vi "Compute 1 A-Scan Parameters.vi"(8 "error in (no error)":errorcluster, 10 "Laser In":refnum<class "Laser.lvclass">, 11 "DAQ Class.lvclass":refnum<class "DAQ Class.lvclass">) -> (0 "error out":errorcluster, 2 "DAQ Parameters":T1, 3 "DAQ Class.lvclass 2":refnum<class "DAQ Class.lvclass">)   [LabVIEW 2015, in "DAQ Class.lvclass"]
uses:
  DAQ Class.lvclass
  DAQ Parameters.ctl
  Trigger Source.ctl
  Trigger Slope.ctl
  Type Defs/OCT DAQ Channel Data Type.ctl
  Clock Control.ctl
  Laser/Laser.lvclass
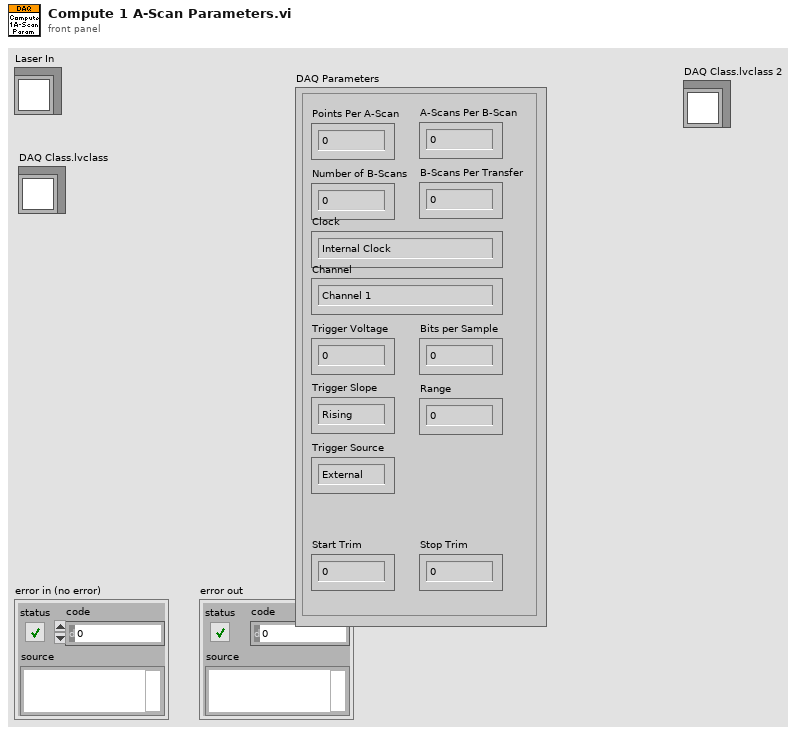
[diagram p1: front panel]
types:
  T1 = typedef "DAQ Class.lvclass/DAQ Parameters.ctl" = cluster{"Points Per A-Scan":u32, "A-Scans Per B-Scan":u32, "Number of B-Scans":u32, "B-Scans Per Transfer":u32, "Trigger Voltage":sgl, "Trigger Source":T2, "Trigger Slope":T3, "Channel":T4, "Clock":T5, "Bits per Sample":dbl, "Range":dbl, "Start Trim":u32, "Stop Trim":u32}
  T2 = typedef "DAQ Class.lvclass/Trigger Source.ctl" = enum16{"External", "Channel A", "Channel B"}
  T3 = typedef "DAQ Class.lvclass/Trigger Slope.ctl" = enum16{"Rising", "Falling"}
  T4 = typedef "OCT DAQ Channel Data Type.ctl" = enum16{"Channel 1", "Channel 2", "Channel 1 and 2"}
  T5 = typedef "DAQ Class.lvclass/Clock Control.ctl" = enum16{"Internal Clock", "External Clock"}
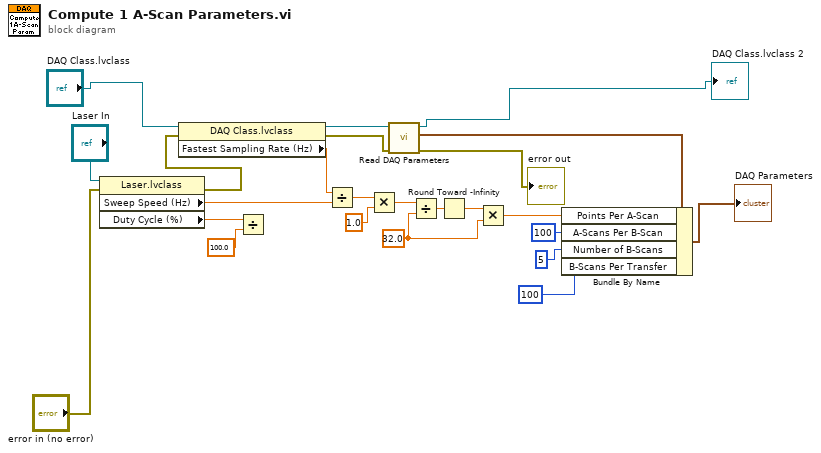
[diagram p0: block diagram]
diagram:
  w22 = 32.0 ("y")
  n1 = property class="Laser.lvclass"(reference="Laser In", error in="error in (no error)") -> (error out=w13:errorcluster, "Sweep Speed (Hz)"=w15:dbl, "Duty Cycle (%)"=w17:dbl)  [unwired: 1 out]
  n2 = property class="DAQ Class.lvclass"(reference="DAQ Class.lvclass", error in=w13) -> (reference out=w6:refnum<class "DAQ Class.lvclass">, error out=w5:errorcluster, "Fastest Sampling Rate (Hz)"=w14:dbl)
  n3 = Divide(x=w17, y=100.0) -> ()  [unwired: 1 out]
  n4 = Divide(x=w14, y=w15) -> (x/y=w16:dbl)
  n5 = Multiply(x=w16, y=1.0) -> (x*y=w19:dbl)
  n6 = call-dynamic "Read DAQ Parameters.vi"("error in (no error)"=w5, "DAQ Class in"=w6) -> ("error out"=→"error out":errorcluster, "DAQ Parameters"=w7:T1, "DAQ Class out"=→"DAQ Class.lvclass 2":refnum<class "DAQ Class.lvclass">)  [unwired: 7 in]
  n7 = Divide(x=w19, y=w22) -> (x/y=w20:dbl)
  n8 = Round Toward -Infinity(1:w20) -> (0:w21:dbl)
  n9 = Multiply(x=w21, y=w22) -> (x*y=w23:dbl)
  n10 = Bundle By Name(cluster=w7, "Points Per A-Scan"=w23, "A-Scans Per B-Scan"=u32 100, "Number of B-Scans"=u32 5, "B-Scans Per Transfer"=u32 100 ("A-Scans Per Transfer")) -> (→"DAQ Parameters":T1)
